vi "Accel to Angles.vi"(1 "accel 2":sgl[](array[numeric]), 2 "accel 1":sgl[](array[numeric])) -> (0 "angles about axis":sgl[](array[numeric]))   [LabVIEW 2010]
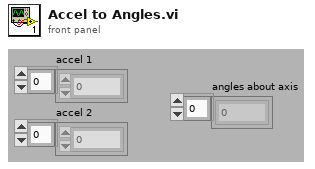
[diagram p1: front panel]
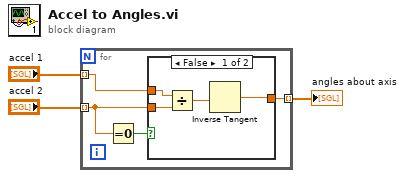
[diagram p0: block diagram]
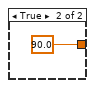
[diagram p2: hidden frame]
diagram:
  n1 = for {
    tunnel: "accel 1" -> [w7] mode=indexing
    tunnel: "accel 2" -> [w6] mode=indexing
    tunnel: [w4] -> w1 mode=indexing
    n2 = Equal To 0?(x=w6) -> (x = 0?=w5:bool)
    n3 = case shown="False" w5 {
      tunnel: w7 -> [w10 _]
      tunnel: w6 -> [w9 _]
      tunnel: [w8 90.0] -> w4
      frame False {
        n4 = Divide(x=w10, y=w9) -> (x/y=w11:sgl)
        n5 = Inverse Tangent(1:w11) -> (0:w8:sgl)
      }
      frame True {
      }
    }
  }
  "angles about axis" <- w1
